vi "BTxtFlash.vi"(6 "BAdress":string, 8 "error in":errorcluster caption="错误输入", 9 "Model":string, 10 "ArrayIn":string[](array[string]), 11 "Path":string="Config\\data.ini") -> (0 "error out":errorcluster caption="错误输出")   [LabVIEW 2013]
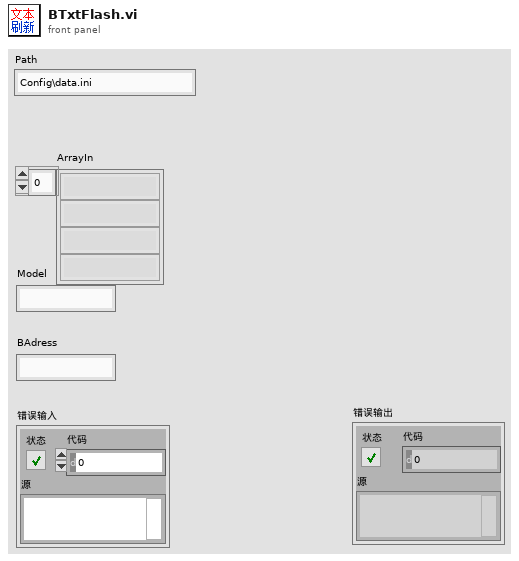
[diagram p1: front panel]
types:
  T1 = enum32{"invalid app kind", "Development System", "Run Time System", "Student Edition", "Embedded LabVIEW", "Evaluation", "Custom"}
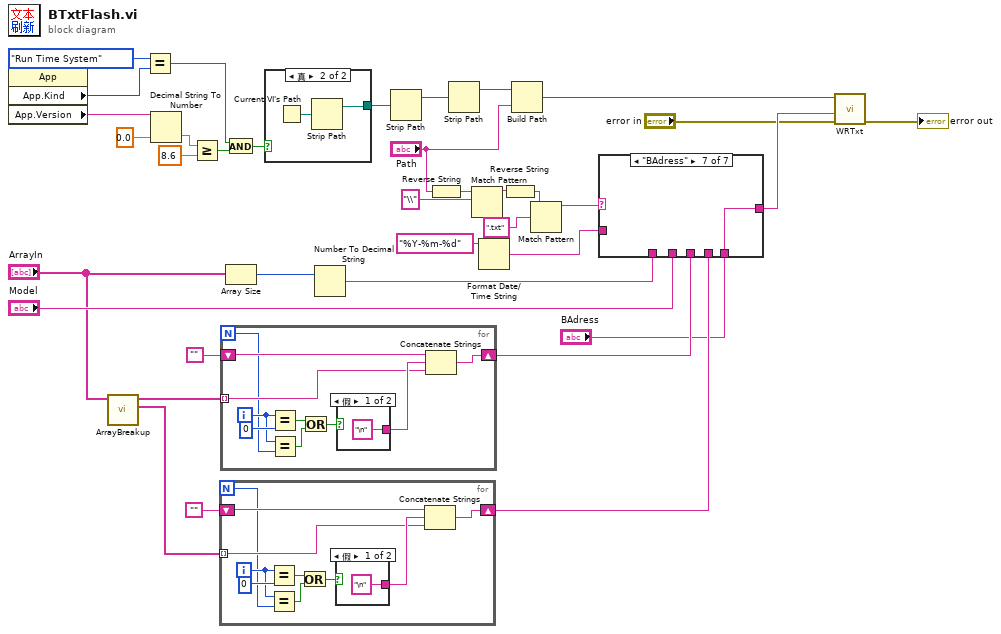
[diagram p0: block diagram]
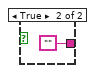
[diagram p2: hidden frame]
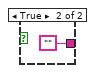
[diagram p3: hidden frame]
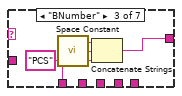
[diagram p6: hidden frame]
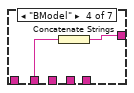
[diagram p7: hidden frame]
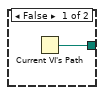
[diagram p10: hidden frame]
diagram:
  n1 = property class="App"() -> ("App.Kind"=w32:T1, "App.Version"=w33:string)  [unwired: 2 in, 2 out]
  n2 = call "ArrayBreakup.vi"("ArrayIn"="ArrayIn") -> ("Array2"=w8:string[], "Array1"=w10:string[])  [unwired: 8 in, 1 out]
  n3 = Equal?(x=T1."Run Time System", y=w32) -> (x = y?=w29:bool)
  n4 = Decimal String To Number(string=w33, default (0L)=0.0 ("y")) -> (number=w35:dbl)  [unwired: 1 in, 1 out]
  n5 = Greater Or Equal?(x=w35, y=8.6) -> (x >= y?=w28:bool)
  n6 = for {
    N -> [w37]
    tunnel: w8 -> [w39] mode=indexing
    shift-right: [w38] -> w7
    shift-left: "" -> [w46]
    i -> [w43]
    n7 = Equal?(x=w43, y=0) -> (x = y?=w45:bool)
    n8 = Equal?(x=w43, y=w37) -> (x = y?=w42:bool)
    n9 = Or(x=w45, y=w42) -> (x .or. y?=w41:bool)
    n10 = case shown="假" w41 {
      tunnel: ["\n" ""] -> w40
      frame False {
      }
      frame True {
      }
    }
    n11 = Concatenate Strings(w46, w40, w39) -> (w38:string)
  }
  n12 = for {
    N -> [w49]
    tunnel: w10 -> [w51] mode=indexing
    shift-right: [w50] -> w13
    shift-left: "" -> [w58]
    i -> [w55]
    n13 = Equal?(x=w55, y=0) -> (x = y?=w57:bool)
    n14 = Equal?(x=w55, y=w49) -> (x = y?=w54:bool)
    n15 = Or(x=w57, y=w54) -> (x .or. y?=w53:bool)
    n16 = case shown="假" w53 {
      tunnel: ["\n" ""] -> w52
      frame False {
      }
      frame True {
      }
    }
    n17 = Concatenate Strings(w58, w52, w51) -> (w50:string)
  }
  n18 = And(x=w29, y=w28) -> (x .and. y?=w30:bool)
  n19 = Array Size(array="ArrayIn") -> (size(s)=w12:i32)
  n20 = case shown="真" w30 {
    tunnel: [w61 w62] -> w26
    frame False {
      n21 = Current VI's Path() -> (path=w61:path)
    }
    frame True {
      n22 = Current VI's Path() -> (path=w63:path)
      n23 = Strip Path(path=w63) -> (stripped path=w62:path)  [unwired: 1 out]
    }
  }
  n24 = Number To Decimal String(number=w12) -> (decimal integer string=w17:string)  [unwired: 1 in]
  n25 = Strip Path(path=w26) -> (stripped path=w25:path)  [unwired: 1 out]
  n26 = Reverse String(1:"Path") -> (0:w4:string)
  n27 = Strip Path(path=w25) -> (stripped path=w27:path)  [unwired: 1 out]
  n28 = Match Pattern(string=w4, regular expression="\\") -> (before substring=w3:string)  [unwired: 1 in, 3 out]
  n29 = Format Date/Time String(time format string (%c)="%Y-%m-%d" ("时间格式字符串(%c)")) -> (date/time string=w20:string)  [unwired: 2 in]
  n30 = Reverse String(1:w3) -> (0:w2:string)
  n31 = Build Path(base path=w27, name or relative path="Path") -> (appended path=w21:path)
  n32 = Match Pattern(string=w2, regular expression=".txt") -> (before substring=w22:string)  [unwired: 1 in, 3 out]
  n33 = case shown="\"BAdress\"" w22 {
    tunnel: w20 -> [_ w64 _ _ _ _ _]
    tunnel: [_ w64 w68 w70 w71 w72 w73] -> w19
    tunnel: w17 -> [_ _ w67 _ _ _ _]
    tunnel: "Model" -> [_ _ _ w69 _ _ _]
    tunnel: w13 -> [_ _ _ _ w71 _ _]
    tunnel: w7 -> [_ _ _ _ _ w72 _]
    tunnel: "BAdress" -> [_ _ _ _ _ _ w73]
    frame "假", Default {
    }
    frame "BDate" {
    }
    frame "BNumber" {
      n34 = call <vilib>:"Space Constant.vi"() -> ("String"=w66:string)
      n35 = Concatenate Strings(w67, w66, "PCS") -> (w68:string)
    }
    frame "BModel" {
      n36 = Concatenate Strings(w69) -> (w70:string)
    }
    frame "BSN1" {
    }
    frame "BSN2" {
    }
    frame "BAdress" {
    }
  }
  n37 = call "WRTxt.vi"("error in"="error in", "Text"=w19, "FilePath"=w21) -> ("error out"=→"error out":errorcluster)  [unwired: 8 in]
